vi "Parse JSON Map.vi"(10 "Name":string, 11 "JSON":string) -> (2 "Found?":bool, 3 "Map":variant)   [LabVIEW 2017]
uses:
  <vilib>/regexp/Match Regular Expression.xnode
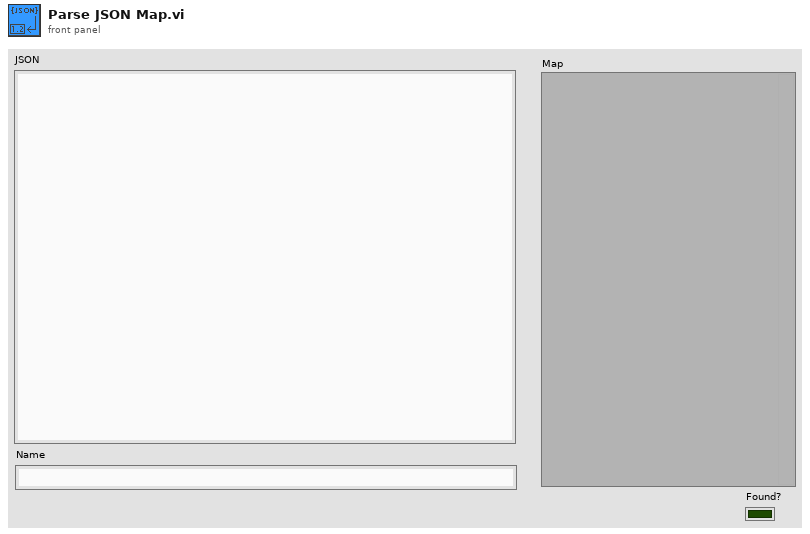
[diagram p1: front panel]
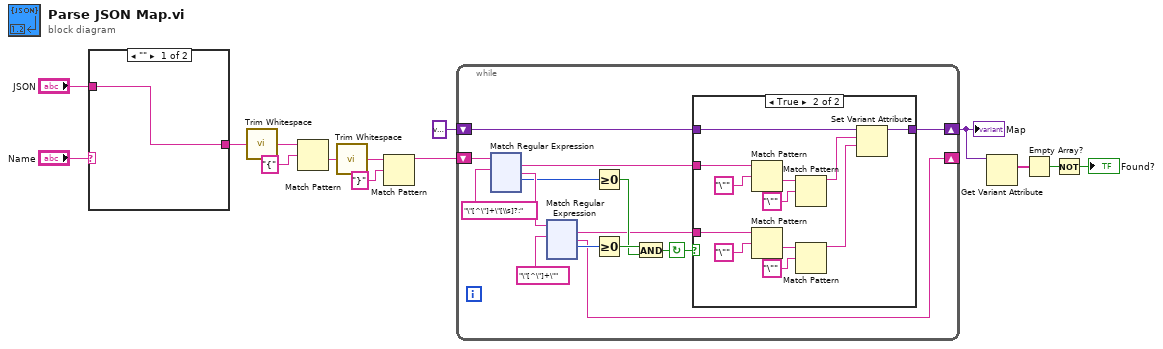
[diagram p0: block diagram]
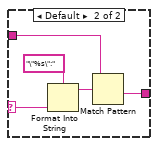
[diagram p2: hidden frame]
diagram:
  n1 = case shown="\"\"" "Name" {
    selector: "Name" -> [_ w16]
    tunnel: [w15 w20] -> w12
    tunnel: "JSON" -> [w15 w17]
    frame "" {
    }
    frame Default {
      n2 = Format Into String(format string="\"%s\":", w16) -> (resulting string=w18:string)  [unwired: 2 in, 1 out]
      n3 = Match Pattern(string=w17, regular expression=w18) -> (after substring=w20:string)  [unwired: 1 in, 3 out]
    }
  }
  n4 = call <vilib>:"Trim Whitespace.vi"("string"=w12) -> ("trimmed string"=w9:string)  [unwired: 1 in]
  n5 = Match Pattern(string=w9, regular expression="{") -> (after substring=w10:string)  [unwired: 1 in, 3 out]
  n6 = call <vilib>:"Trim Whitespace.vi"("string"=w10) -> ("trimmed string"=w8:string)  [unwired: 1 in]
  n7 = Match Pattern(string=w8, regular expression="}") -> (before substring=w14:string)  [unwired: 1 in, 3 out]
  n8 = while {
    shift-right: [w21] -> _
    shift-left: w14 -> [w34]
    shift-right: [w24] -> w4
    shift-left: variant -> [w25]
    stop <- w26 continue-if-true
    n9 = xnode "Match Regular Expression"("input string"=w34, "regular expression"="\"[^\"]+\"[\\s]?:") -> ("whole match"=w28:string, "after match"=w33:string, "offset past match"=w29:i32)  [unwired: 4 in, 2 out]
    n10 = xnode "Match Regular Expression"("input string"=w33, "regular expression"="\"[^\"]+\"") -> ("whole match"=w27:string, "after match"=w21:string, "offset past match"=w32:i32)  [unwired: 4 in, 2 out]
    n11 = Greater Or Equal To 0?(x=w29) -> (x >= 0?=w30:bool)
    n12 = Greater Or Equal To 0?(x=w32) -> (x >= 0?=w31:bool)
    n13 = And(x=w31, y=w30) -> (x .and. y?=w26:bool)
    n14 = case shown="True" w26 {
      tunnel: w28 -> [_ w44]
      tunnel: w27 -> [_ w40]
      tunnel: w25 -> [w35 w39]
      tunnel: [w35 w38] -> w24
      frame False {
      }
      frame True {
        n15 = Match Pattern(string=w44, regular expression="\"") -> (after substring=w45:string)  [unwired: 1 in, 3 out]
        n16 = Match Pattern(string=w40, regular expression="\"") -> (after substring=w43:string)  [unwired: 1 in, 3 out]
        n17 = Match Pattern(string=w45, regular expression="\"") -> (before substring=w37:string)  [unwired: 1 in, 3 out]
        n18 = Match Pattern(string=w43, regular expression="\"") -> (before substring=w36:string)  [unwired: 1 in, 3 out]
        n19 = Set Variant Attribute(Variant=w39, name=w37, value=w36) -> (Variant out=w38:variant)  [unwired: 1 in, 2 out]
      }
    }
  }
  "Map" <- w4
  n20 = Get Variant Attribute(Variant=w4) -> (names=w3:string[])  [unwired: 3 in, 3 out]
  n21 = Empty Array?(array=w3) -> (empty?=w2:bool)
  n22 = Not(x=w2) -> (.not. x?=→"Found?":bool)
